vi "Chain3.vi"(7 "Name (\"\" to Use UUID)":string="CSM-Module") -> ()   [LabVIEW 2017, in "CSM-Testcase.lvlib"]
doc: "Creates a template for a CSM module without a user interface.\n\n> [!NOTE] CSM Name Rules\n> - The CSM module name must be unique to avoid entering the \"Critical Error\" state.\n> - If the input is \"\", a UUID will be used as the module name. This module will operate in independent mode and will not be listed in the module list.\n> - If the input ends with '#', the module will run in work mode. Modules with the same name will share the same message queue. External messages will be handled by the idle module.\n\n> [!NOTE] CSM Initialization State\n> - The default value is \"Macro: Initialize\", consistent with the JKISM state machine.\n> - This state is typically not modified and is provided to facilitate external programmatic changes to the initialization state.\n\n\n-- <b>Controls</b> --\n- <b>Name (\"\" to Use UUID)</b>: CSM Module Name\n- <b>Init State(\"Macro: Initialize\")</b>: Initialization State, default is \"Macro: Initialize\""
uses:
  CSM-Testcase.lvlib
  src/user.lib/_NEVSTOP/Communicable State Machine(CSM)/AdvanceAPI/CSM - Revert Arguments-Safe String.vi
  src/user.lib/_NEVSTOP/Communicable State Machine(CSM)/AdvanceAPI/CSM - Make String Arguments Safe.vi
  src/user.lib/_NEVSTOP/Communicable State Machine(CSM)/AdvanceAPI/CSM - Break Down Multiple States String.vi
  src/user.lib/_NEVSTOP/Communicable State Machine(CSM)/AdvanceAPI/CSM - Keywords.vi
  src/user.lib/_NEVSTOP/Communicable State Machine(CSM)/_Shared/Trim Single-line Text.vi
  Global-TestcaseCSM.vi
  src/user.lib/_NEVSTOP/Communicable State Machine(CSM)/_Polymophic/Build No-Reply Asynchronous Message with Arguments.vi
  src/user.lib/_NEVSTOP/Communicable State Machine(CSM)/_Polymophic/Build Asynchronous Message with Arguments.vi
  src/user.lib/_NEVSTOP/Communicable State Machine(CSM)/_Polymophic/Build Register Message.vi
  src/user.lib/_NEVSTOP/Communicable State Machine(CSM)/_Polymophic/Build Interrupt Broadcast Message.vi
  src/user.lib/_NEVSTOP/Communicable State Machine(CSM)/Communicable State Machine.lvlib
panel:
  out "Error Occurred":errorcluster
  out "State History":string
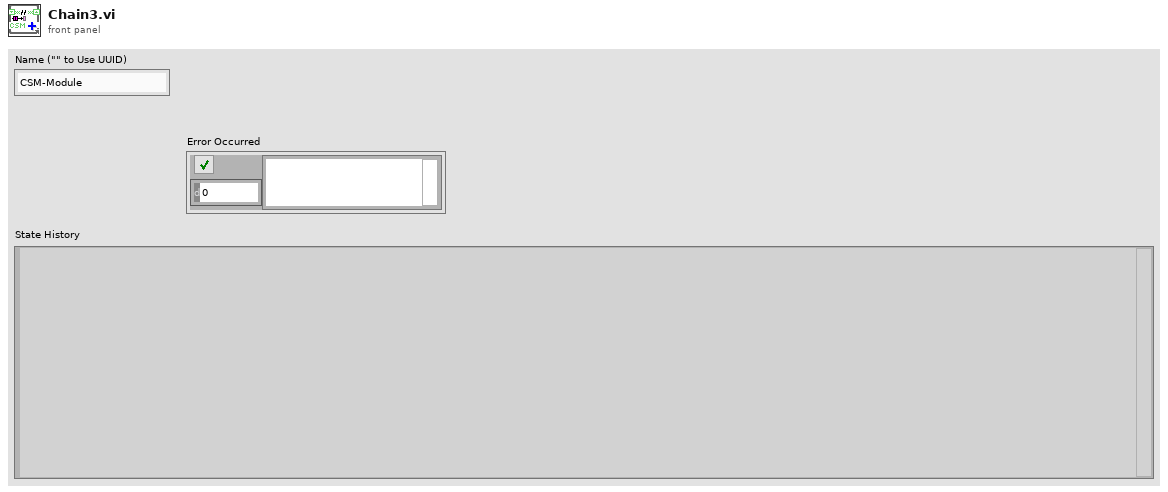
[diagram p1: front panel]
types:
  T1 = cluster{"Arguments":string, "Response":string, "error":errorcluster}
  T2 = enum32{"Invalid", "Standard", "Closed", "Hidden", "Minimized", "Maximized"}
  T3 = enum32{"invalid app kind", "Development System", "Run Time System", "Student Edition", "Embedded LabVIEW", "Evaluation", "Custom"}
  T4 = typedef "Communicable State Machine.lvlib/_CSM_Response Source Message.ctl" = cluster{"‘State":string, "’Arguments":string, "’Error":errorcluster}
  T5 = cluster{"Current VI Reference":refnum<vi>, "Close Panel on Exit?":bool}
  T6 = cluster{"Core":cluster{"Current VI Reference":refnum<vi>, "Close Panel on Exit?":bool}, "Your Boolean data":bool, "Your string data":string, "Counter":u32}
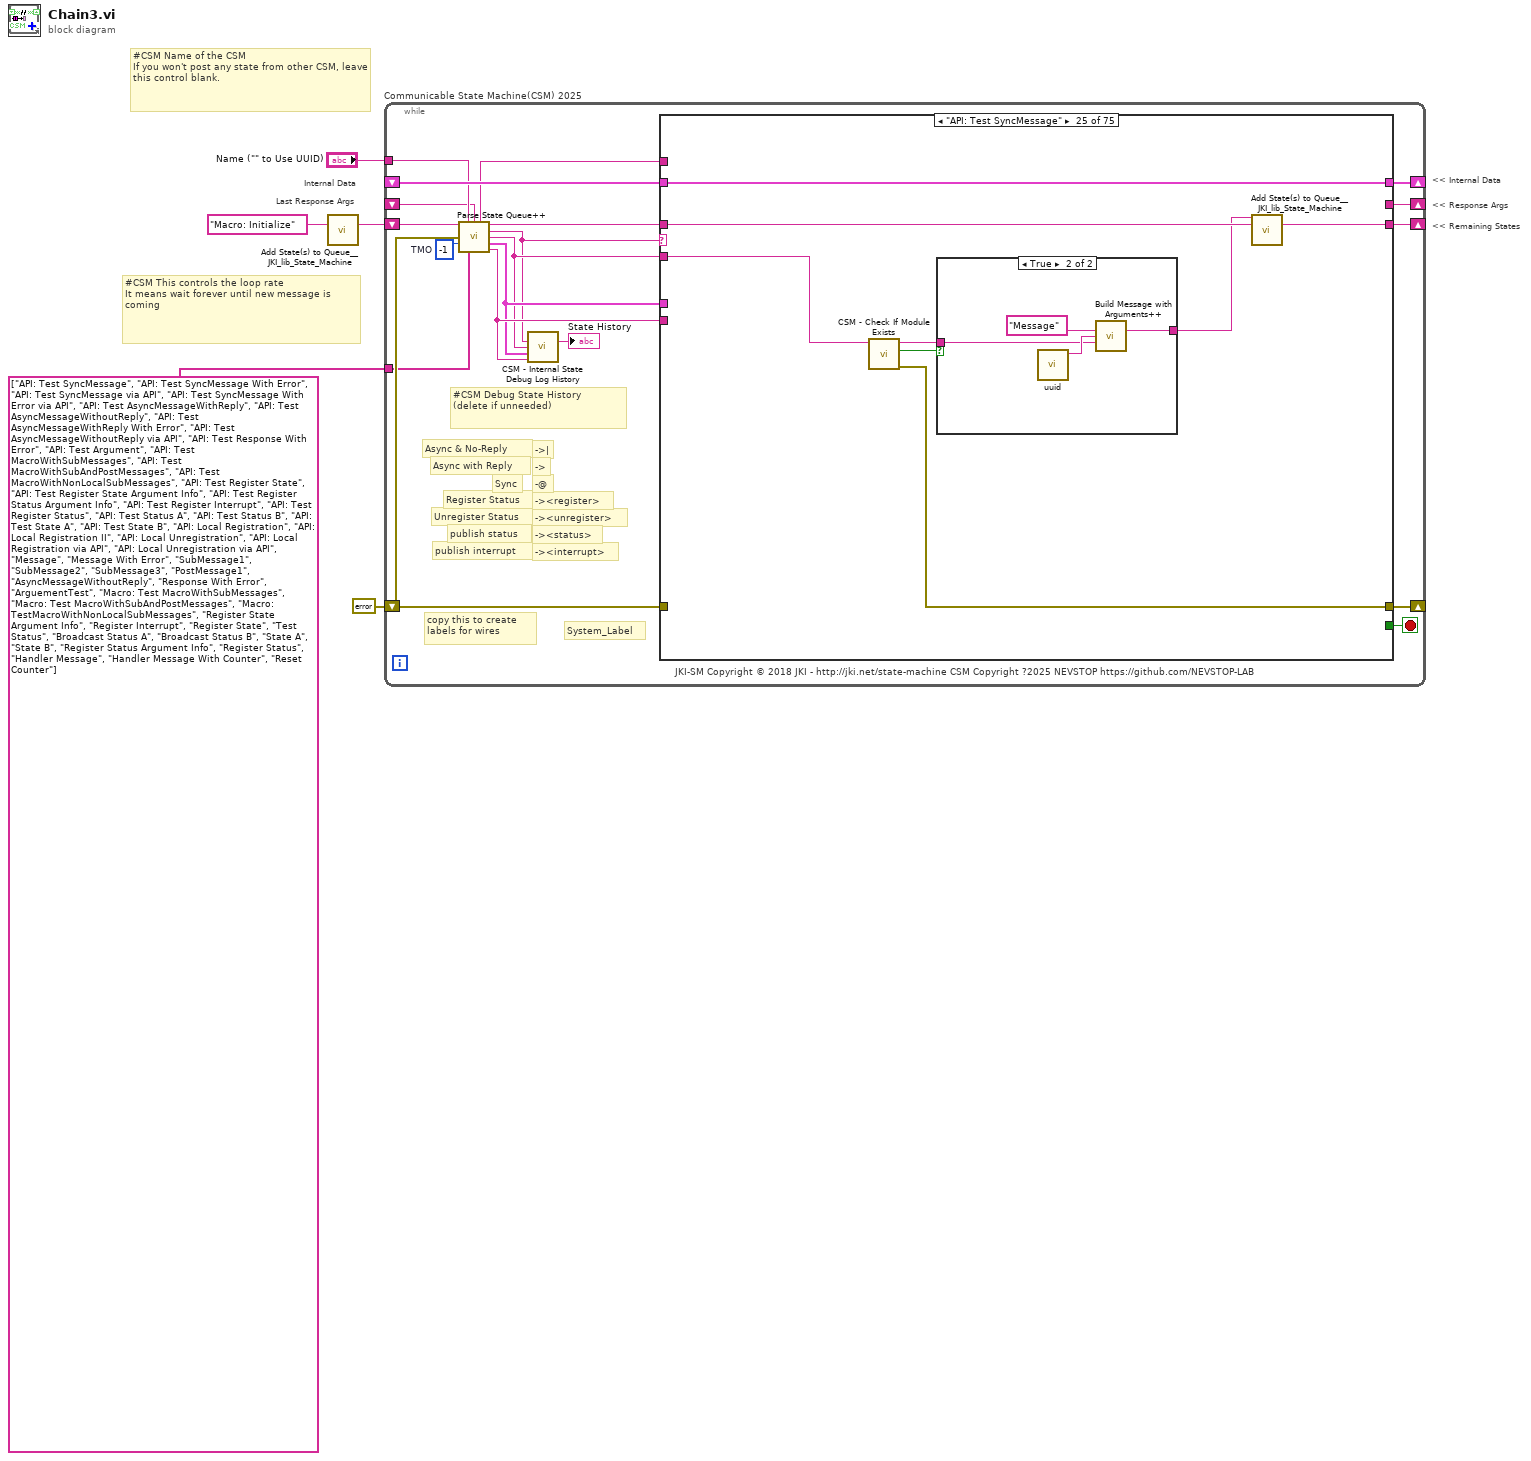
[diagram p0: block diagram]
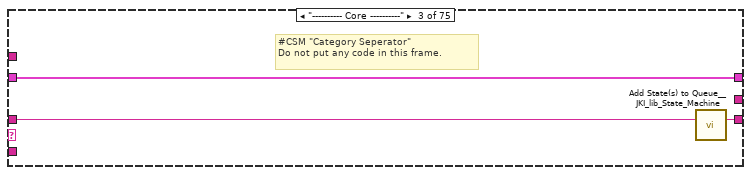
[diagram p4: hidden frame]
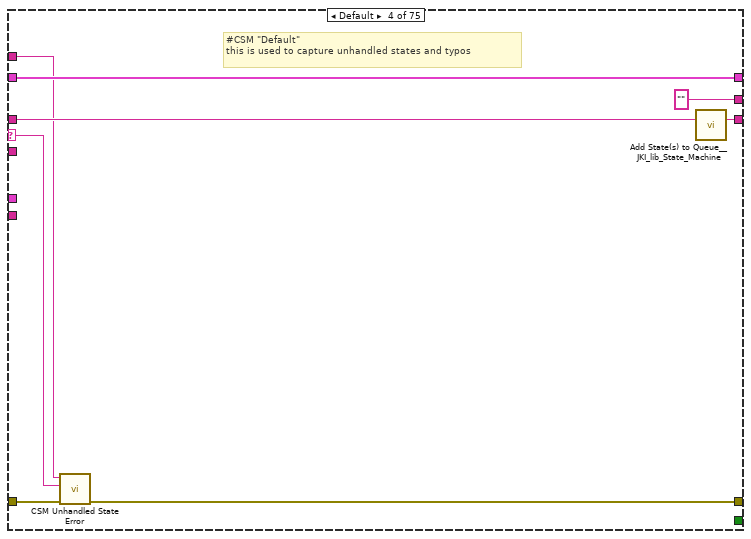
[diagram p5: hidden frame]
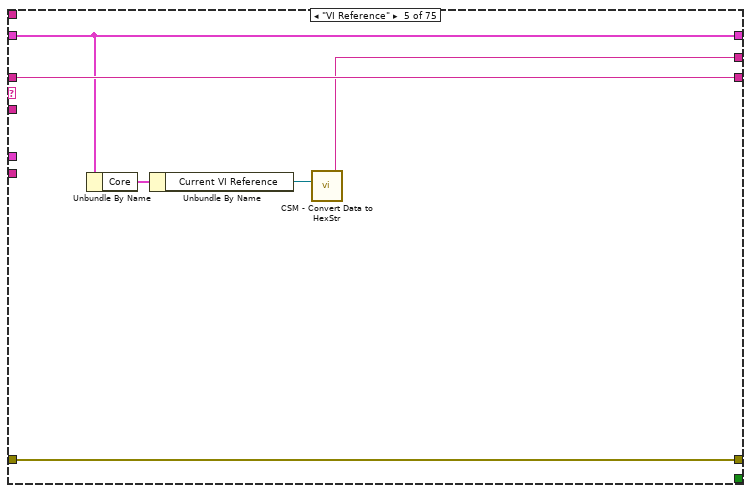
[diagram p6: hidden frame]
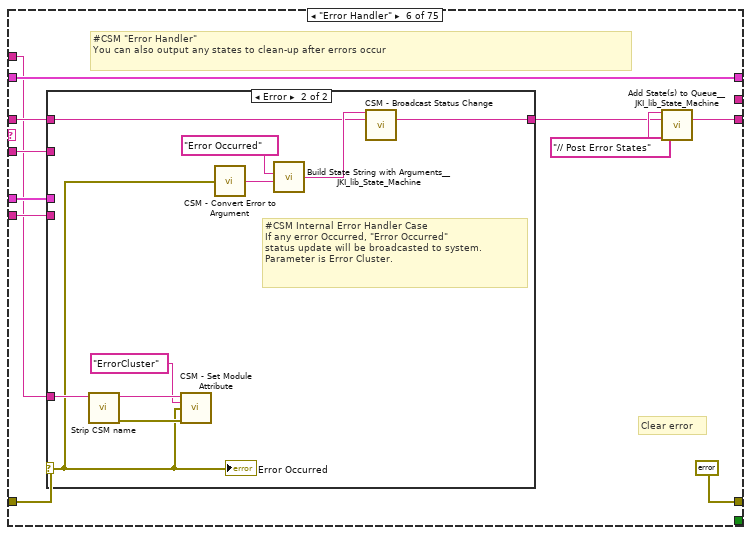
[diagram p7: hidden frame]
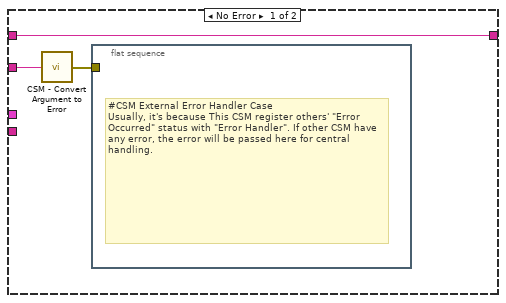
[diagram p8: hidden frame]
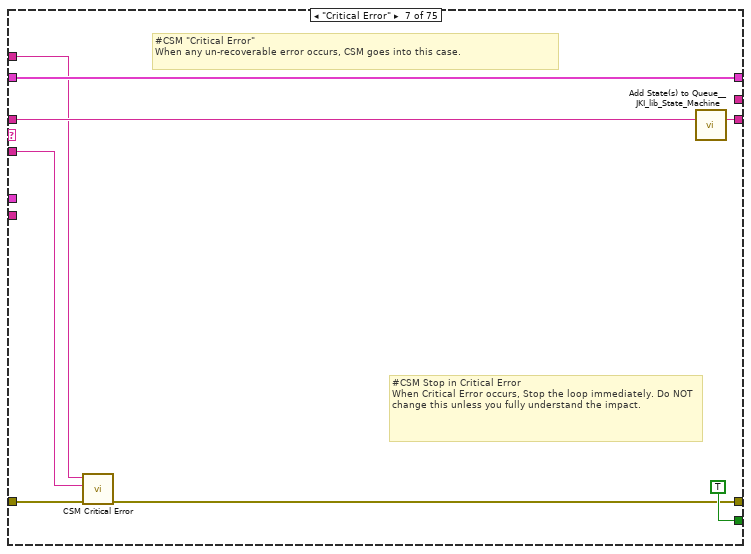
[diagram p9: hidden frame]
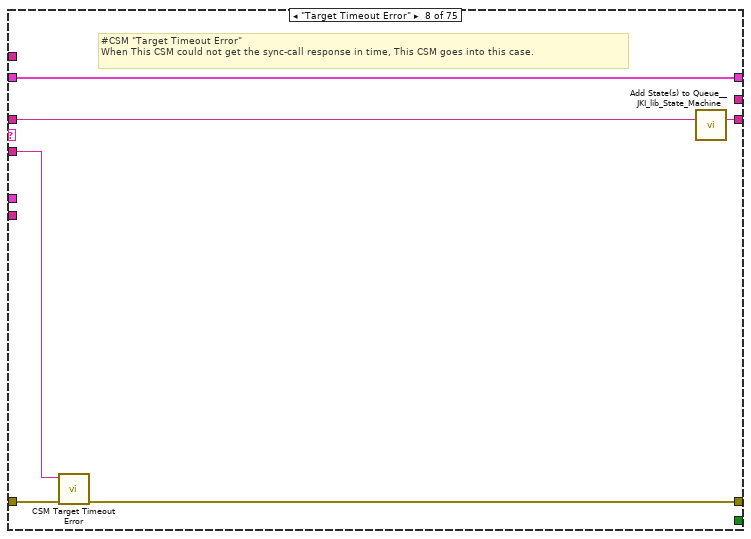
[diagram p10: hidden frame]
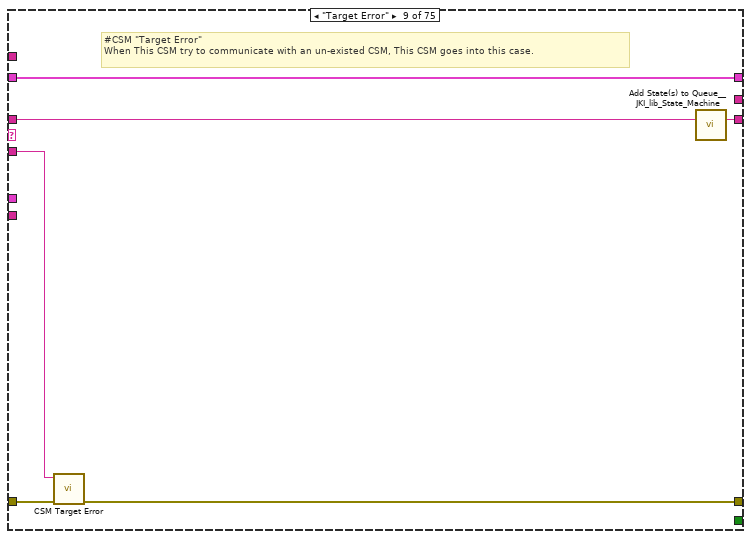
[diagram p11: hidden frame]
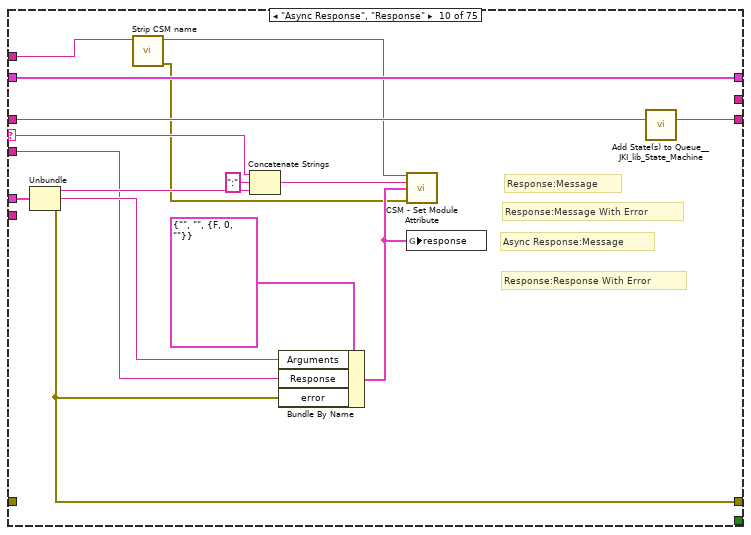
[diagram p12: hidden frame]
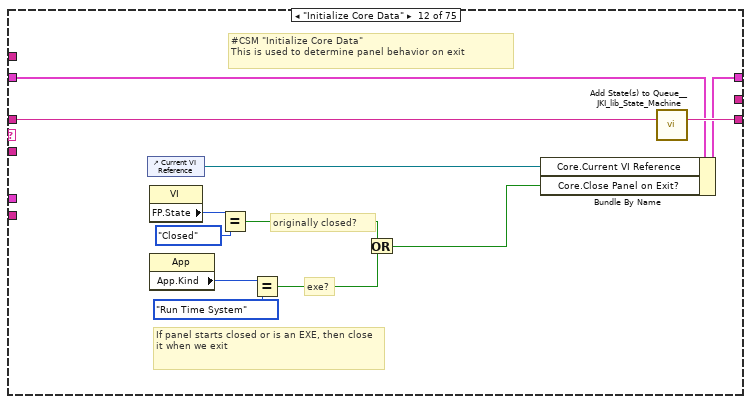
[diagram p14: hidden frame]
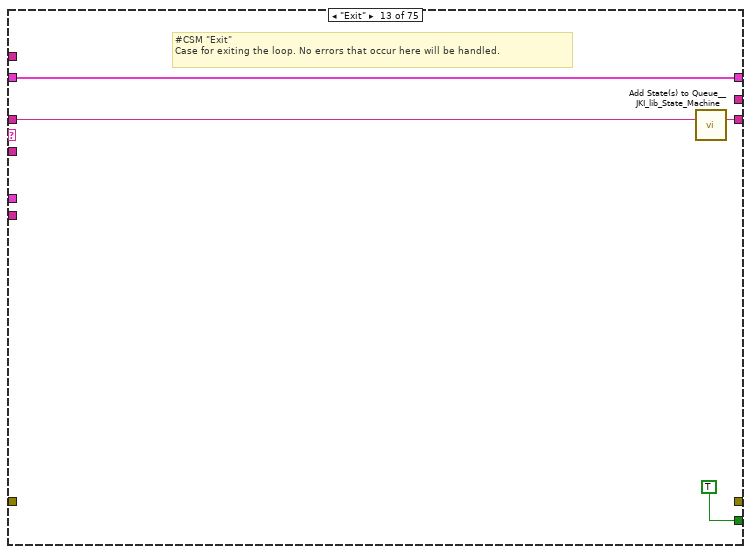
[diagram p15: hidden frame]
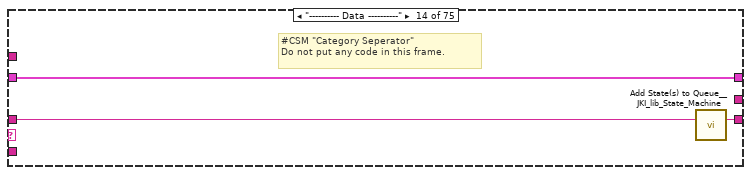
[diagram p16: hidden frame]
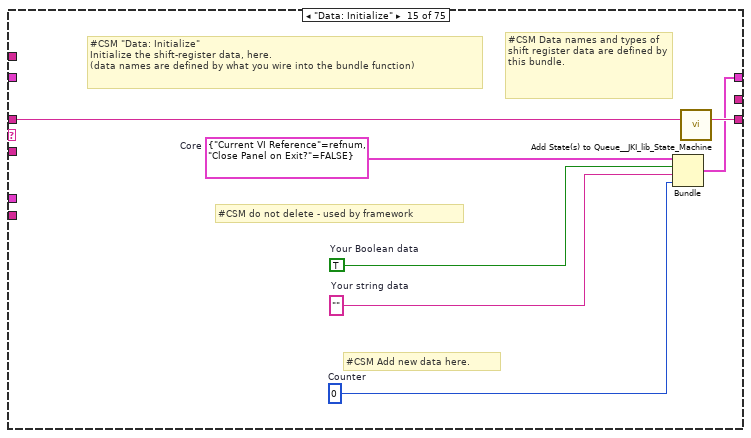
[diagram p17: hidden frame]
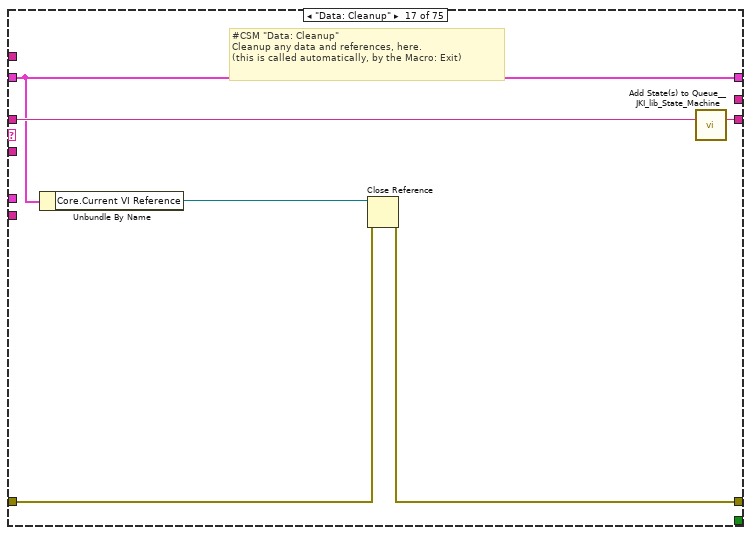
[diagram p19: hidden frame]
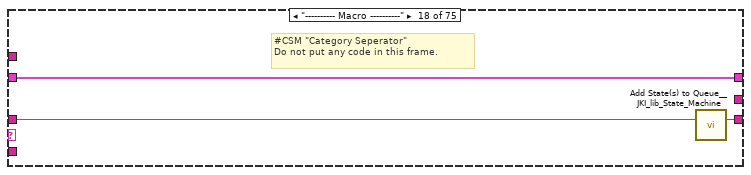
[diagram p20: hidden frame]
diagram:
  # "Last Response Args"
  # "Internal Data"
  # "#CSM Name of the CSM\nIf you won't post any state from other CSM, leave this control blank."
  # "#CSM This controls the loop rate\nIt means wait forever until new message is coming"
  # "<< Internal Data"
  # "<< Response Args"
  # "<< Remaining States"
  n1 = call <vilib>:"Add State(s) to Queue__JKI_lib_State_Machine.vi"("State(s) in (\"\")"="Macro: Initialize" ("Init State(\"Macro: Initialize\")")) -> ("States Out"=w5:string)  [unwired: 14 in]
  n2 = while "Communicable State Machine(CSM) 2025" {
    shift-right: [w19] -> _
    shift-left: _ -> [w18]
    shift-right: [w22] -> _
    shift-left: errorcluster {"status"=FALSE, "code"=0, "source"=""} ("error out") -> [w8]
    shift-right: [w21] -> _
    shift-left: w5 -> [w23]
    tunnel: "Name (\"\" to Use UUID)" -> [w15]
    shift-right: [w16] -> _
    shift-left: _ -> [w10]
    tunnel: string[] ["API: Test SyncMessage", "API: Test SyncMessage With Error", "API: Test SyncMessage via API", "API: Test SyncMessage With Error via API", "API: Test AsyncMessageWithReply", "API: Test AsyncMessageWithoutReply", "API: Test AsyncMessageWithReply With Error", "API: Test AsyncMessageWithoutReply via API", "API: Test Response With Error", "API: Test Argument", "API: Test MacroWithSubMessages", "API: Test MacroWithSubAndPostMessages", "API: Test MacroWithNonLocalSubMessages", "API: Test Register State", "API: Test Register State Argument Info", "API: Test Register Status Argument Info", "API: Test Register Interrupt", "API: Test Register Status", "API: Test Status A", "API: Test Status B", "API: Test State A", "API: Test State B", "API: Local Registration", "API: Local Registration II", "API: Local Unregistration", "API: Local Registration via API", "API: Local Unregistration via API", "Message", "Message With Error", "SubMessage1", "SubMessage2", "SubMessage3", "PostMessage1", "AsyncMessageWithoutReply", "Response With Error", "ArguementTest", "Macro: Test MacroWithSubMessages", "Macro: Test MacroWithSubAndPostMessages", "Macro: TestMacroWithNonLocalSubMessages", "Register State Argument Info", "Register Interrupt", "Register State", "Test Status", "Broadcast Status A", "Broadcast Status B", "State A", "State B", "Register Status Argument Info", "Register Status", "Handler Message", "Handler Message With Counter", "Reset Counter"] ("Allowed Messages (Empty for All)") -> [w6]
    stop <- w20 stop-if-true
    w17 = -1  # TMO
    # "#CSM Debug State History\n(delete if unneeded)"
    # "-><interrupt>"
    # "-><status>"
    # "-><unregister>"
    # "-><register>"
    # "-@"
    # "->"
    # "->|"
    # "publish interrupt"
    # "publish status"
    # "Unregister Status"
    # "Register Status"
    # "Sync"
    # "Async with Reply"
    # "Async & No-Reply"
    # "JKI-SM Copyright © 2018 JKI - http://jki.net/state-machine CSM Copyright ?2025 NEVSTOP https://github.com/NEVSTOP-LAB"
    # "copy this to create labels for wires"
    # "System_Label"
    n3 = call "Parse State Queue++.vi"("State Queue"=w23, "Name (\"\" to Use UUID)"=w15, "Response Arguments"=w10, "Previous Error"=w8, "Dequeue (1 ms)"=w17, "Allowed Messages (Empty for All)"=w6) -> ("Name Used"=w9:string, "Remaining States"=w24:string, "Current State"=w11:string, "Arguments"=w12:string, "Additional Information"=w13:T4, "Source CSM"=w14:string)  [unwired: 4 in]
    n4 = call "CSM - Internal State Debug Log History.vi"("State"=w11, "Arguments (\"\")"=w12, ">> Response Source Message >>"=w13, "Source (\"\")"=w14) -> ("Debug Log"=→"State History":string)  [unwired: 11 in]
    n5 = case shown="\"API: Test SyncMessage\"" w11 {
      selector: w11 -> [_ _ _ w35 _ _ _ _ _ w101 _ _ _ _ _ _ _ _ _ _ _ _ _ _ _ _ _ _ _ _ _ _ _ _ _ _ _ _ _ _ _ _ _ _ _ _ _ _ _ _ _ _ _ _ _ w543 _ _ _ _ _ _ _ _ _ _ w611 _ _ _ w636 w649 w656 w672 _]
      tunnel: w24 -> [w25 w28 w31 w39 w44 w50 w77 w83 w89 w105 w107 w119 w123 w126 w133 w135 w141 w144 w148 w154 w168 w188 w217 w221 w225 w237 w265 w297 w313 w325 w337 w351 w374 w385 w398 w405 w412 w419 w426 w433 w440 w447 w454 w461 w468 w475 w487 w496 w506 w516 w526 w530 w535 w538 w542 w549 w556 w559 w572 w578 w584 w588 w593 w597 w601 w605 w615 w619 w627 w633 w641 w651 w661 w677 w689]
      tunnel: w12 -> [_ _ _ _ _ w49 w73 w80 w86 w95 _ _ _ _ _ _ _ _ _ _ w155 w175 w200 _ w228 w240 w268 w300 w316 w328 w340 w354 w370 w388 w395 w402 w409 w416 w423 w430 w437 w444 w451 w458 w465 w472 w479 _ w498 w507 w517 w528 _ _ w539 _ w552 w561 _ w574 w580 w586 w591 w596 w600 w604 w610 w618 w625 w631 w638 w650 w655 w667 _]
      tunnel: w18 -> [w26 w27 w29 w37 w43 w55 w75 w81 w87 w103 w106 w113 w121 w124 _ w134 w136 w142 w146 w152 w170 w190 w219 w220 w229 w241 w269 w301 w317 w329 w341 w355 w377 w389 w400 w407 w414 w421 w428 w435 w442 w449 w456 w463 w470 w477 w485 w494 w504 w514 w524 w529 w533 w536 w540 w550 w557 w563 w573 w579 w585 w590 w595 w598 w602 w606 w616 w620 w626 w632 w642 w652 w662 w669 w687]
      tunnel: [_ _ _ w32 w45 errorcluster {"status"=FALSE, "code"=0, "source"=""} ("error out") w70 w78 w84 w94 _ _ _ _ _ _ w137 _ _ _ _ _ _ _ w222 w234 w262 w294 w310 w322 w334 w347 w371 w382 w399 w406 w413 w420 w427 w434 w441 w448 w455 w462 w469 w476 w481 w490 w500 w511 w521 _ _ _ _ w545 _ _ w565 _ _ w589 w594 w599 w603 w607 w609 w621 w622 w628 w635 w645 w657 w673 _] -> w22
      tunnel: w8 -> [_ _ _ w33 w45 w53 w71 w79 w85 _ _ _ _ _ _ _ w138 _ _ _ _ _ _ _ _ _ _ _ _ _ _ _ _ _ w399 w406 w413 w420 w427 w434 w441 w448 w455 w462 w469 w476 _ _ _ _ _ _ _ _ _ _ _ _ _ _ _ w589 w594 w599 w603 w607 w617 w621 w623 w629 w643 w653 w663 w678 _]
      tunnel: [w25 w28 w30 w38 w44 w51 w76 w82 w88 w104 w107 w118 w122 w125 w132 w135 w140 w143 w147 w153 w169 w189 w218 w221 w226 w238 w266 w298 w314 w326 w338 w352 w375 w386 w397 w404 w411 w418 w425 w432 w439 w446 w453 w460 w467 w474 w486 w495 w505 w515 w525 w530 w534 w537 w541 w551 w553 w558 w570 w575 w581 w587 w592 w597 w601 w605 w615 w619 w627 w633 w641 w651 w661 w677 w688] -> w21
      tunnel: [_ _ _ _ _ _ TRUE _ _ _ _ _ TRUE _ _ _ _ _ _ _ _ _ _ _ _ _ _ _ _ _ _ _ _ _ _ _ _ _ _ _ _ _ _ _ _ _ _ _ _ _ _ _ _ _ _ _ _ _ _ _ _ _ _ _ _ _ _ _ _ _ _ _ _ _ _] -> w20
      tunnel: [w26 w27 w29 w37 w43 w55 w75 w81 w87 w103 w106 w117 w121 w124 w131 w134 w136 w142 w146 w152 w170 w190 w219 w220 w229 w241 w269 w301 w317 w329 w341 w355 w377 w389 w400 w407 w414 w421 w428 w435 w442 w449 w456 w463 w470 w477 w485 w494 w504 w514 w524 w529 w533 w536 w540 w550 w557 w563 w573 w579 w585 w590 w595 w598 w602 w606 w616 w620 w626 w632 w642 w652 w662 w668 w685] -> w19
      tunnel: w14 -> [_ _ _ _ _ w48 _ _ _ _ _ _ _ _ _ _ _ _ _ _ _ _ _ _ _ _ _ _ _ _ _ _ _ _ _ _ _ _ _ _ _ _ _ _ _ _ _ _ _ _ _ _ _ _ _ _ _ _ _ _ _ _ _ _ _ _ _ _ _ _ _ _ _ _ _]
      tunnel: w13 -> [_ _ _ _ _ w47 _ _ _ w102 _ _ _ _ _ _ _ _ _ _ _ _ _ _ _ _ _ _ _ _ _ _ _ _ _ _ _ _ _ _ _ _ _ _ _ _ _ _ _ _ _ _ _ _ _ _ _ _ _ _ _ _ _ _ _ _ _ _ _ _ _ _ _ _ _]
      tunnel: [_ _ _ "" w40 _ _ _ _ _ _ _ _ _ _ _ _ _ _ _ _ _ _ _ _ _ _ _ _ _ _ _ _ _ _ _ _ _ _ _ _ _ _ _ _ _ _ _ _ _ _ w527 _ _ w539 w544 _ _ _ _ _ w586 w591 w596 w600 w604 w610 w618 w625 w631 _ w650 w655 _ _] -> w16
      tunnel: w9 -> [_ _ _ w34 _ w46 w72 _ _ w92 _ _ _ _ _ _ _ _ _ _ _ _ _ _ _ _ w253 w285 _ _ _ w348 _ _ _ _ _ _ _ _ _ _ _ _ _ _ w483 w492 w502 w513 w523 _ _ _ _ w546 _ _ w567 _ _ _ _ _ _ _ w614 _ _ _ w640 w648 w660 w676 _]
      frame "", "Idle" {
        # "#CSM \"Idle/Event Handler\"\nexecutes when the state queue is empty"
      }
      frame "CSM Documentation" {
        # "#CSM State Syntax\n\n// Comment line, all text to the right of “//” will be ignored\n// Local Message Example\nDoSth: DoA >> Arguments\n\n// Sync Call Example\nAPI: xxxx >> Arguments -@ TargetModule\n\n// Async Call Example\nAPI: xxxx >> Arguments -> TargetModule\n\n// Async Call without Reply Example\nAPI: xxxx >> Arguments ->| TargetModule\n\n// Broadcast normal status:\nStatus >> StatusArguments  -><status>\n\n// Broadcast Interrupt status:\nInterrupt >> StatusArguments  -><interrupt>\n\n// Register Source Module's status to Handler Module\nStatus@Source Module >> Handler Module@Handler Module -><register>\n\n// Unegister Source Module's status\nStatus@Source Module >> Handler Module -><unregister>"
        # "#CSM README FIRST\n\nCommunicable State Machine(CSM) is a LabVIEW application framework that builds upon JKI State Machine(JKISM). It follows the pattern of JKISM and extends the keywords to describe message communication between modules, including concepts such as Sync-Message, Async-Message, Subscription/Unsubscription of status - essential elements for creating reusable code modules. For more information, please visit the CSM wiki: https://nevstop-lab.github.io/CSM-Wiki/\n\nFor instructions on JKI State Machine, visit: \n    http://jki.net/state-machine/\nFor information about CSM, visit: \n    https://github.com/NEVSTOP-LAB"
        # "#CSM \"Documentation\"\nCase for holding CSM Documenation"
      }
      frame "---------- Core ----------" {
        # "#CSM \"Category Seperator\"\nDo not put any code in this frame."
        n6 = call <vilib>:"Add State(s) to Queue__JKI_lib_State_Machine.vi"("State(s) in (\"\")"=w31) -> ("States Out"=w30:string)  [unwired: 14 in]
      }
      frame Default {
        # "#CSM \"Default\"\nthis is used to capture unhandled states and typos"
        n7 = call "CSM Unhandled State Error.vi"("error in (no error)"=w33, "Undefined State"=w35, "CSM Name"=w34) -> ("error out"=w32:errorcluster)  [unwired: 8 in]
        n8 = call <vilib>:"Add State(s) to Queue__JKI_lib_State_Machine.vi"("State(s) in (\"\")"=w39) -> ("States Out"=w38:string)  [unwired: 14 in]
      }
      frame "VI Reference" {
        n9 = Unbundle By Name(w43) -> ("Core"=w42:T5)
        n10 = Unbundle By Name(w42) -> ("Current VI Reference"=w41:refnum<vi>)
        n11 = call "CSM - Convert Data to HexStr.vi"("Variant"=w41) -> ("HEX String (0-9,A-F)"=w40:string)  [unwired: 8 in]
      }
      frame "Error Handler" {
        # "#CSM \"Error Handler\"\nYou can also output any states to clean-up after errors occur"
        # "Clear error"
        n12 = case shown="Error" w53 {
          selector: w53 -> [_ w61]
          tunnel: [w59 w66] -> w52
          tunnel: w50 -> [w59 w65]
          tunnel: w49 -> [w58 _]
          tunnel: w48 -> [_ _]
          tunnel: w47 -> [_ _]
          tunnel: w46 -> [_ w64]
          frame No Error {
            n13 = call "CSM - Convert Argument to Error.vi"("Argument"=w58) -> ("Error"=w57:errorcluster)  [unwired: 4 in]
            n14 = flat-sequence {
              tunnel: w57 -> [_]
              frame #0 {
                # "#CSM External Error Handler Case\nUsually, it's because This CSM register others' \"Error Occurred\" status with \"Error Handler\". If other CSM have any error, the error will be passed here for central handling."
              }
            }
          }
          frame Error {
            # "#CSM Internal Error Handler Case \nIf any error Occurred, \"Error Occurred\" \nstatus update will be broadcasted to system.\nParameter is Error Cluster."
            n15 = call "Strip CSM name.vi"("CSM name"=w64) -> ("error out"=w63:errorcluster, "CSM name core"=w62:string)  [unwired: 7 in, 2 out]
            n16 = call "CSM - Set Module Attribute.vi"("CSM Name"=w62, "Attribute"="ErrorCluster", "Value"=w61, "Error In"=w63) -> ()  [unwired: 8 in, 4 out]
            n17 = call "CSM - Convert Error to Argument.vi"("Error"=w61) -> ("Argument"=w68:string)  [unwired: 4 in]
            n18 = call <vilib>:"Build State String with Arguments__JKI_lib_State_Machine.vi"("Arguments (\"\")"=w68, "State"="Error Occurred" ("Status with Arguments")) -> ("State with Arguments"=w67:string)  [unwired: 4 in]
            n19 = call "CSM - Broadcast Status Change.vi"("Status With Arguments"=w67, "State Queue"=w65) -> ("Remaining States"=w66:string)  [unwired: 13 in]
            "Error Occurred" <- w61
          }
        }
        n20 = call <vilib>:"Add State(s) to Queue__JKI_lib_State_Machine.vi"("State(s) in Front (\"\")"="// Post Error States", "State(s) in (\"\")"=w52) -> ("States Out"=w51:string)  [unwired: 13 in]
      }
      frame "Critical Error" {
        # "#CSM \"Critical Error\"\nWhen any un-recoverable error occurs, CSM goes into this case."
        # "#CSM Stop in Critical Error\nWhen Critical Error occurs, Stop the loop immediately. Do NOT change this unless you fully understand the impact."
        n21 = call "CSM Critical Error.vi"("error in (no error)"=w71, "Arugments (As Reason)"=w73, "CSM Name"=w72) -> ("error out"=w70:errorcluster)  [unwired: 8 in]
        n22 = call <vilib>:"Add State(s) to Queue__JKI_lib_State_Machine.vi"("State(s) in (\"\")"=w77) -> ("States Out"=w76:string)  [unwired: 14 in]
      }
      frame "Target Timeout Error" {
        # "#CSM \"Target Timeout Error\"\nWhen This CSM could not get the sync-call response in time, This CSM goes into this case."
        n23 = call "CSM Target Timeout Error.vi"("error in (no error)"=w79, "Arguments (As CSM Name)"=w80) -> ("error out"=w78:errorcluster)  [unwired: 9 in]
        n24 = call <vilib>:"Add State(s) to Queue__JKI_lib_State_Machine.vi"("State(s) in (\"\")"=w83) -> ("States Out"=w82:string)  [unwired: 14 in]
      }
      frame "Target Error" {
        # "#CSM \"Target Error\"\nWhen This CSM try to communicate with an un-existed CSM, This CSM goes into this case."
        n25 = call "CSM Target Error.vi"("error in (no error)"=w85, "Arguments (As CSM Name)"=w86) -> ("error out"=w84:errorcluster)  [unwired: 9 in]
        n26 = call <vilib>:"Add State(s) to Queue__JKI_lib_State_Machine.vi"("State(s) in (\"\")"=w89) -> ("States Out"=w88:string)  [unwired: 14 in]
      }
      frame "Async Response", "Response" {
        # "Response:Response With Error"
        # "Response:Message With Error"
        # "Async Response:Message"
        # "Response:Message"
        n27 = Unbundle(w102) -> ("‘State"=w100:string, "’Arguments"=w96:string, "’Error"=w94:errorcluster)
        n28 = call "Strip CSM name.vi"("CSM name"=w92) -> ("error out"=w90:errorcluster, "CSM name core"=w91:string)  [unwired: 7 in, 2 out]
        n29 = Concatenate Strings(w101, ":" ("string"), w100) -> (w98:string)
        n30 = Bundle By Name(cluster=T1 {"Arguments"="", "Response"="", "error"={"status"=FALSE, "code"=0, "source"=""}}, "Arguments"=w96, "Response"=w95, "error"=w94) -> (w93:T1)
        n31 = call "CSM - Set Module Attribute.vi"("CSM Name"=w91, "Attribute"=w98, "Value"=w93, "Error In"=w90) -> ()  [unwired: 8 in, 4 out]
        n32 = global write "Global-TestcaseCSM.vi" "response"(w93) -> ()
        n33 = call <vilib>:"Add State(s) to Queue__JKI_lib_State_Machine.vi"("State(s) in (\"\")"=w105) -> ("States Out"=w104:string)  [unwired: 14 in]
      }
      frame "Async Message Posted" {
        # "#CSM \"Async Message Posted\"\nAfter Async Message is posted (-> or ->| ), CSM goes to this state for post-action.\nYou can use Argument - State to tell which Async Message is called."
      }
      frame "Initialize Core Data" {
        # "#CSM \"Initialize Core Data\"\nThis is used to determine panel behavior on exit"
        # "originally closed?"
        # "exe?"
        # "If panel starts closed or is an EXE, then close it when we exit"
        n34 = control-ref of="Current VI Reference"() -> (w111:refnum<vi>)
        n35 = property class="VI"() -> ("FP.State"=w110:T2)  [unwired: 2 in, 2 out]
        n36 = property class="App"() -> ("App.Kind"=w116:T3)  [unwired: 2 in, 2 out]
        n37 = Equal?(x=w110, y=T2."Closed" ("Front Panel Window:State")) -> (x = y?=w108:bool)
        n38 = Equal?(x=w116, y=T3."Run Time System" ("Application:Kind")) -> (x = y?=w114:bool)
        n39 = Or(x=w108, y=w114) -> (x .or. y?=w112:bool)
        n40 = Bundle By Name(cluster=w113, "Core.Current VI Reference"=w111, "Core.Close Panel on Exit?"=w112) -> (w117:T6)
        n41 = call <vilib>:"Add State(s) to Queue__JKI_lib_State_Machine.vi"("State(s) in (\"\")"=w119) -> ("States Out"=w118:string)  [unwired: 14 in]
      }
      frame "Exit" {
        # "#CSM \"Exit\"\nCase for exiting the loop. No errors that occur here will be handled."
        n42 = call <vilib>:"Add State(s) to Queue__JKI_lib_State_Machine.vi"("State(s) in (\"\")"=w123) -> ("States Out"=w122:string)  [unwired: 14 in]
      }
      frame "---------- Data ----------" {
        # "#CSM \"Category Seperator\"\nDo not put any code in this frame."
        n43 = call <vilib>:"Add State(s) to Queue__JKI_lib_State_Machine.vi"("State(s) in (\"\")"=w126) -> ("States Out"=w125:string)  [unwired: 14 in]
      }
      frame "Data: Initialize" {
        w127 = u32 0  # Counter
        w128 = T5 {"Current VI Reference"=refnum, "Close Panel on Exit?"=FALSE}  # Core
        w130 = TRUE  # Your Boolean data
        w129 = ""  # Your string data
        # "#CSM \"Data: Initialize\"\nInitialize the shift-register data, here.\n(data names are defined by what you wire into the bundle function)"
        # "#CSM do not delete - used by framework"
        # "#CSM Add new data here."
        # "#CSM Data names and types of shift register data are defined by this bundle."
        n44 = Bundle("Core"=w128, "Your Boolean data"=w130, "Your string data"=w129, "Counter"=w127) -> (w131:T6)  [unwired: 1 in]
        n45 = call <vilib>:"Add State(s) to Queue__JKI_lib_State_Machine.vi"("State(s) in (\"\")"=w133) -> ("States Out"=w132:string)  [unwired: 14 in]
      }
      frame "Data: Update Indicators" {
      }
      frame "Data: Cleanup" {
        # "#CSM \"Data: Cleanup\"\nCleanup any data and references, here.\n(this is called automatically, by the Macro: Exit)"
        n46 = Unbundle By Name(w136) -> ("Core.Current VI Reference"=w139:refnum<vi>)
        n47 = Close Reference(reference=w139, error in (no error)=w138) -> (error out=w137:errorcluster)
        n48 = call <vilib>:"Add State(s) to Queue__JKI_lib_State_Machine.vi"("State(s) in (\"\")"=w141) -> ("States Out"=w140:string)  [unwired: 14 in]
      }
      frame "---------- Macro ----------" {
        # "#CSM \"Category Seperator\"\nDo not put any code in this frame."
        n49 = call <vilib>:"Add State(s) to Queue__JKI_lib_State_Machine.vi"("State(s) in (\"\")"=w144) -> ("States Out"=w143:string)  [unwired: 14 in]
      }
      frame "Macro: Initialize" {
        # "#CSM \"Macro: Initialize\"\nInitialization Macro (This is called once, when the VI starts)"
        n50 = call <vilib>:"Add State(s) to Queue__JKI_lib_State_Machine.vi"("State(s) in Front (\"\")"="Data: Initialize\nInitialize Core Data\nData: Update Indicators", "State(s) in (\"\")"=w148) -> ("States Out"=w147:string)  [unwired: 13 in]
      }
      frame "Macro: Exit" {
        # "#CSM \"Macro: Exit\"\nExit Macro (This is called once, when the VI exits)"
        n51 = call <vilib>:"Add State(s) to Queue__JKI_lib_State_Machine.vi"("State(s) in Front (\"\")"="//Exit Sub-Modules ", "State(s) at Back (\"\")"="Data: Cleanup\nExit") -> ("States Out"=w150:string)  [unwired: 13 in]
        n52 = call <vilib>:"Add State(s) to Queue__JKI_lib_State_Machine.vi"("State(s) in Front (\"\")"=w150, "State(s) in (\"\")"=w154) -> ("States Out"=w153:string)  [unwired: 13 in]
      }
      frame "Macro: Test MacroWithSubMessages" {
        w156 = "SubMessage2" ("State With Arguments")
        w158 = "SubMessage1" ("State With Arguments")
        n53 = call "uuid.vi"() -> ("UUID"=w157:string)  [unwired: 11 in]
        n54 = call "uuid.vi"() -> ("UUID"=w159:string)  [unwired: 11 in]
        n55 = Concatenate Strings(w158, w159) -> (w160:string)
        n56 = Concatenate Strings(w156, w157) -> (w161:string)
        n57 = call <vilib>:"Build State String with Arguments__JKI_lib_State_Machine.vi"("Arguments (\"\")"=w155, "State"="SubMessage3" ("State With Arguments")) -> ("State with Arguments"=w163:string)  [unwired: 4 in]
        n58 = call <vilib>:"Build State String with Arguments__JKI_lib_State_Machine.vi"("Arguments (\"\")"=w160, "State"=w158) -> ("State with Arguments"=w165:string)  [unwired: 4 in]
        n59 = call <vilib>:"Build State String with Arguments__JKI_lib_State_Machine.vi"("Arguments (\"\")"=w161, "State"=w156) -> ("State with Arguments"=w164:string)  [unwired: 4 in]
        n60 = Build Array(w165, w164, w163) -> (w162:string[])
        n61 = call "CSM - Compact Multiple States.vi"("Multiple States"=w162) -> ("States"=w167:string)  [unwired: 9 in]
        n62 = call <vilib>:"Add State(s) to Queue__JKI_lib_State_Machine.vi"("State(s) in Front (\"\")"=w167, "State(s) in (\"\")"=w168) -> ("States Out"=w169:string)  [unwired: 13 in]
      }
      frame "Macro: Test MacroWithSubAndPostMessages" {
        w174 = "PostMessage1" ("State With Arguments")
        w176 = "SubMessage2" ("State With Arguments")
        w178 = "SubMessage1" ("State With Arguments")
        n63 = call "uuid.vi"() -> ("UUID"=w177:string)  [unwired: 11 in]
        n64 = call "uuid.vi"() -> ("UUID"=w173:string)  [unwired: 11 in]
        n65 = call "uuid.vi"() -> ("UUID"=w179:string)  [unwired: 11 in]
        n66 = Concatenate Strings(w174, w173) -> (w172:string)
        n67 = Concatenate Strings(w178, w179) -> (w180:string)
        n68 = Concatenate Strings(w176, w177) -> (w181:string)
        n69 = call <vilib>:"Build State String with Arguments__JKI_lib_State_Machine.vi"("Arguments (\"\")"=w175, "State"="SubMessage3" ("State With Arguments")) -> ("State with Arguments"=w183:string)  [unwired: 4 in]
        n70 = call <vilib>:"Build State String with Arguments__JKI_lib_State_Machine.vi"("Arguments (\"\")"=w172, "State"=w174) -> ("State with Arguments"=w171:string)  [unwired: 4 in]
        n71 = call <vilib>:"Build State String with Arguments__JKI_lib_State_Machine.vi"("Arguments (\"\")"=w180, "State"=w178) -> ("State with Arguments"=w185:string)  [unwired: 4 in]
        n72 = call <vilib>:"Build State String with Arguments__JKI_lib_State_Machine.vi"("Arguments (\"\")"=w181, "State"=w176) -> ("State with Arguments"=w184:string)  [unwired: 4 in]
        n73 = Build Array(w185, w184, w183) -> (w182:string[])
        n74 = call "CSM - Compact Multiple States.vi"("Multiple States"=w182) -> ("States"=w187:string)  [unwired: 9 in]
        n75 = call <vilib>:"Add State(s) to Queue__JKI_lib_State_Machine.vi"("State(s) in Front (\"\")"=w187, "State(s) in (\"\")"=w188, "State(s) at Back (\"\")"=w171) -> ("States Out"=w189:string)  [unwired: 12 in]
      }
      frame "Macro: TestMacroWithNonLocalSubMessages" {
        w204 = "PostMessage1" ("State With Arguments")
        w205 = "SubMessage2" ("State With Arguments")
        w207 = "SubMessage1" ("State With Arguments")
        n76 = Match Pattern(string=w200, regular expression="+") -> (before substring=w192:string, after substring=w191:string)  [unwired: 1 in, 2 out]
        n77 = call "uuid.vi"() -> ("UUID"=w203:string)  [unwired: 11 in]
        n78 = call "uuid.vi"() -> ("UUID"=w206:string)  [unwired: 11 in]
        n79 = call "uuid.vi"() -> ("UUID"=w208:string)  [unwired: 11 in]
        n80 = Concatenate Strings(w204, w203) -> (w202:string)
        n81 = Concatenate Strings(w207, w208) -> (w209:string)
        n82 = Concatenate Strings(w205, w206) -> (w210:string)
        n83 = call <vilib>:"Build State String with Arguments__JKI_lib_State_Machine.vi"("Arguments (\"\")"=w202, "State"=w204) -> ("State with Arguments"=w201:string)  [unwired: 4 in]
        n84 = call-poly "Build Message with Arguments++.vi"("State With Arguments"="SubMessage1", "Target Module (\"\")"=w191) -> ("CSM Message String"=w196:string)  [unwired: 13 in]
        n85 = call-poly "Build Message with Arguments++.vi"("State With Arguments"="SubMessage2", "Target Module (\"\")"=w191) -> ("CSM Message String"=w195:string)  [unwired: 13 in]
        n86 = call <vilib>:"Build State String with Arguments__JKI_lib_State_Machine.vi"("Arguments (\"\")"=w192, "State"="SubMessage3" ("State With Arguments")) -> ("State with Arguments"=w212:string)  [unwired: 4 in]
        n87 = call-poly "Build Message with Arguments++.vi"("State With Arguments"="Message", "Target Module (\"\")"=w191) -> ("CSM Message String"=w197:string)  [unwired: 13 in]
        n88 = call <vilib>:"Build State String with Arguments__JKI_lib_State_Machine.vi"("Arguments (\"\")"=w209, "State"=w207) -> ("State with Arguments"=w214:string)  [unwired: 4 in]
        n89 = call <vilib>:"Build State String with Arguments__JKI_lib_State_Machine.vi"("Arguments (\"\")"=w210, "State"=w205) -> ("State with Arguments"=w213:string)  [unwired: 4 in]
        n90 = Build Array(w214, w213, w212, w197, w196, w195) -> (w211:string[])
        n91 = call "CSM - Compact Multiple States.vi"("Multiple States"=w211) -> ("States"=w216:string)  [unwired: 9 in]
        n92 = call <vilib>:"Add State(s) to Queue__JKI_lib_State_Machine.vi"("State(s) in Front (\"\")"=w216, "State(s) in (\"\")"=w217, "State(s) at Back (\"\")"=w201) -> ("States Out"=w218:string)  [unwired: 12 in]
      }
      frame "---------- API ----------" {
        # "#CSM \"Category Seperator\"\nDo not put any code in this frame."
      }
      frame "API: Test SyncMessage" {
        n93 = call "CSM - Check If Module Exists.vi"("CSM Name"=w228) -> ("error out"=w222:errorcluster, "Exist?"=w223:bool, "CSM Name (Dup)"=w227:string)  [unwired: 8 in]
        n94 = case shown="True" w223 {
          tunnel: w227 -> [_ w231]
          tunnel: [_ w230] -> w224
          frame False {
          }
          frame True {
            n95 = call "uuid.vi"() -> ("UUID"=w232:string)  [unwired: 11 in]
            n96 = call-poly "Build Message with Arguments++.vi"("State With Arguments"="Message", "Arguments (\"\")"=w232, "Target Module (\"\")"=w231) -> ("CSM Message String"=w230:string)  [unwired: 12 in]
          }
        }
        n97 = call <vilib>:"Add State(s) to Queue__JKI_lib_State_Machine.vi"("State(s) in Front (\"\")"=w224, "State(s) in (\"\")"=w225) -> ("States Out"=w226:string)  [unwired: 13 in]
      }
      frame "API: Test SyncMessage With Error" {
        n98 = call "CSM - Check If Module Exists.vi"("CSM Name"=w240) -> ("error out"=w234:errorcluster, "Exist?"=w235:bool, "CSM Name (Dup)"=w239:string)  [unwired: 8 in]
        n99 = case shown="True" w235 {
          tunnel: w239 -> [_ w243]
          tunnel: [_ w242] -> w236
          frame False {
          }
          frame True {
            n100 = call "uuid.vi"() -> ("UUID"=w244:string)  [unwired: 11 in]
            n101 = call "Build Synchronous Message with Arguments.vi"("State With Arguments"="Message With Error", "Arguments (\"\")"=w244, "Target Module (\"\")"=w243) -> ("CSM Message String"=w242:string)  [unwired: 12 in]
          }
        }
        n102 = call <vilib>:"Add State(s) to Queue__JKI_lib_State_Machine.vi"("State(s) in Front (\"\")"=w236, "State(s) in (\"\")"=w237) -> ("States Out"=w238:string)  [unwired: 13 in]
      }
      frame "API: Test SyncMessage via API" {
        n103 = call "CSM - Check If Module Exists.vi"("CSM Name"=w268) -> ("error out"=w263:errorcluster, "Exist?"=w264:bool, "CSM Name (Dup)"=w267:string)  [unwired: 8 in]
        n104 = case shown="True" w264 {
          tunnel: w267 -> [_ w277]
          tunnel: [_ w276] -> w251
          tunnel: w253 -> [_ w275]
          tunnel: [_ w274] -> w260
          tunnel: [_ w273] -> w249
          tunnel: [_ w272] -> w256
          tunnel: [_ w271] -> w259
          frame False {
          }
          frame True {
            w274 = "Message" ("State With Arguments")
            n105 = call "uuid.vi"() -> ("UUID"=w272:string)  [unwired: 11 in]
            n106 = call "CSM - Wait and Send Message for Reply.vi"("State"=w274, "Current Module (\"\" to Generate an ID)"=w275, "Arguments (\"\")"=w272, "Target Module"=w277) -> ("Response"=w271:string, "Source CSM"=w273:string, "error out"=w276:errorcluster)  [unwired: 9 in]
          }
        }
        n107 = call "Strip CSM name.vi"("CSM name"=w253) -> ("error out"=w250:errorcluster, "CSM name core"=w252:string)  [unwired: 7 in, 2 out]
        n108 = call "Strip CSM name.vi"("CSM name"=w249) -> ("error out"=w246:errorcluster, "CSM name core"=w248:string)  [unwired: 7 in, 2 out]
        n109 = Bundle By Name(cluster=T1 {"Arguments"="", "Response"="", "error"={"status"=FALSE, "code"=0, "source"=""}}, "Arguments"=w256, "Response"=w259, "error"=w251) -> (w254:T1)
        n110 = Concatenate Strings(w248, ":" ("string"), w260) -> (w258:string)
        n111 = Merge Errors(w250, w246) -> (w247:errorcluster)
        n112 = call "CSM - Set Module Attribute.vi"("CSM Name"=w252, "Attribute"=w258, "Value"=w254, "Error In"=w247) -> ("error out"=w257:errorcluster)  [unwired: 8 in, 3 out]
        n113 = disable-structure shown="Enabled" {
          disable-tunnel: w254 -> [w270 _]
          frame Enabled {
            n114 = global write "Global-TestcaseCSM.vi" "response"(w270) -> ()
          }
          frame Disabled {
          }
        }
        n115 = call <vilib>:"Add State(s) to Queue__JKI_lib_State_Machine.vi"("State(s) in (\"\")"=w265) -> ("States Out"=w266:string)  [unwired: 14 in]
        n116 = Merge Errors(w257, w251, w263) -> (w262:errorcluster)
      }
      frame "API: Test SyncMessage With Error via API" {
        n117 = call "CSM - Check If Module Exists.vi"("CSM Name"=w300) -> ("error out"=w295:errorcluster, "Exist?"=w296:bool, "CSM Name (Dup)"=w299:string)  [unwired: 8 in]
        n118 = case shown="True" w296 {
          tunnel: w299 -> [_ w309]
          tunnel: [_ w308] -> w282
          tunnel: w285 -> [_ w307]
          tunnel: [_ w306] -> w292
          tunnel: [_ w305] -> w281
          tunnel: [_ w304] -> w288
          tunnel: [_ w303] -> w291
          frame False {
          }
          frame True {
            w306 = "Message With Error" ("State With Arguments")
            n119 = call "uuid.vi"() -> ("UUID"=w304:string)  [unwired: 11 in]
            n120 = call "CSM - Wait and Send Message for Reply.vi"("State"=w306, "Current Module (\"\" to Generate an ID)"=w307, "Arguments (\"\")"=w304, "Target Module"=w309) -> ("Response"=w303:string, "Source CSM"=w305:string, "error out"=w308:errorcluster)  [unwired: 9 in]
          }
        }
        n121 = call "Strip CSM name.vi"("CSM name"=w281) -> ("error out"=w278:errorcluster, "CSM name core"=w280:string)  [unwired: 7 in, 2 out]
        n122 = Bundle By Name(cluster=T1 {"Arguments"="", "Response"="", "error"={"status"=FALSE, "code"=0, "source"=""}}, "Arguments"=w288, "Response"=w291, "error"=w282) -> (w287:T1)
        n123 = call "Strip CSM name.vi"("CSM name"=w285) -> ("error out"=w283:errorcluster, "CSM name core"=w284:string)  [unwired: 7 in, 2 out]
        n124 = Concatenate Strings(w280, ":" ("string"), w292) -> (w290:string)
        n125 = Merge Errors(w283, w278) -> (w279:errorcluster)
        n126 = disable-structure shown="Enabled" {
          disable-tunnel: w287 -> [w302 _]
          frame Enabled {
            n127 = global write "Global-TestcaseCSM.vi" "response"(w302) -> ()
          }
          frame Disabled {
          }
        }
        n128 = call "CSM - Set Module Attribute.vi"("CSM Name"=w284, "Attribute"=w290, "Value"=w287, "Error In"=w279) -> ("error out"=w289:errorcluster)  [unwired: 8 in, 3 out]
        n129 = call <vilib>:"Add State(s) to Queue__JKI_lib_State_Machine.vi"("State(s) in (\"\")"=w297) -> ("States Out"=w298:string)  [unwired: 14 in]
        n130 = Merge Errors(w289, w282, w295) -> (w294:errorcluster)
      }
      frame "API: Test AsyncMessageWithReply" {
        n131 = call "CSM - Check If Module Exists.vi"("CSM Name"=w316) -> ("error out"=w310:errorcluster, "Exist?"=w311:bool, "CSM Name (Dup)"=w315:string)  [unwired: 8 in]
        n132 = case shown="True" w311 {
          tunnel: w315 -> [_ w319]
          tunnel: [_ w318] -> w312
          frame False {
          }
          frame True {
            n133 = call "uuid.vi"() -> ("UUID"=w320:string)  [unwired: 11 in]
            n134 = call-poly "Build Message with Arguments++.vi"("State With Arguments"="Message", "Arguments (\"\")"=w320, "Target Module (\"\")"=w319) -> ("CSM Message String"=w318:string)  [unwired: 12 in]
          }
        }
        n135 = call <vilib>:"Add State(s) to Queue__JKI_lib_State_Machine.vi"("State(s) in Front (\"\")"=w312, "State(s) in (\"\")"=w313) -> ("States Out"=w314:string)  [unwired: 13 in]
      }
      frame "API: Test AsyncMessageWithReply With Error" {
        n136 = call "CSM - Check If Module Exists.vi"("CSM Name"=w328) -> ("error out"=w322:errorcluster, "Exist?"=w323:bool, "CSM Name (Dup)"=w327:string)  [unwired: 8 in]
        n137 = case shown="True" w323 {
          tunnel: w327 -> [_ w332]
          tunnel: [_ w330] -> w324
          frame False {
          }
          frame True {
            n138 = call "uuid.vi"() -> ("UUID"=w331:string)  [unwired: 11 in]
            n139 = call-poly "Build Message with Arguments++.vi"("State With Arguments"="Message With Error", "Arguments (\"\")"=w331, "Target Module (\"\")"=w332) -> ("CSM Message String"=w330:string)  [unwired: 12 in]
          }
        }
        n140 = call <vilib>:"Add State(s) to Queue__JKI_lib_State_Machine.vi"("State(s) in Front (\"\")"=w324, "State(s) in (\"\")"=w325) -> ("States Out"=w326:string)  [unwired: 13 in]
      }
      frame "API: Test AsyncMessageWithoutReply" {
        n141 = call "CSM - Check If Module Exists.vi"("CSM Name"=w340) -> ("error out"=w334:errorcluster, "Exist?"=w335:bool, "CSM Name (Dup)"=w339:string)  [unwired: 8 in]
        n142 = case shown="True" w335 {
          tunnel: w339 -> [_ w345]
          tunnel: [_ w343] -> w336
          frame False {
          }
          frame True {
            n143 = call-poly "Build Message with Arguments++.vi"("State With Arguments"="AsyncMessageWithoutReply", "Arguments (\"\")"="123456789" ("Arguments (\"\")"), "Target Module (\"\")"=w345) -> ("CSM Message String"=w343:string)  [unwired: 12 in]
          }
        }
        n144 = call <vilib>:"Add State(s) to Queue__JKI_lib_State_Machine.vi"("State(s) in Front (\"\")"=w336, "State(s) in (\"\")"=w337) -> ("States Out"=w338:string)  [unwired: 13 in]
      }
      frame "API: Test AsyncMessageWithoutReply via API" {
        n145 = call "CSM - Check If Module Exists.vi"("CSM Name"=w354) -> ("error out"=w349:errorcluster, "Exist?"=w350:bool, "CSM Name (Dup)"=w353:string)  [unwired: 8 in]
        n146 = case shown="True" w350 {
          tunnel: w353 -> [_ w357]
          tunnel: w348 -> [_ w360]
          tunnel: [_ w356] -> w346
          frame False {
          }
          frame True {
            n147 = call "CSM - Wait and Post Message.vi"("State"="AsyncMessageWithoutReply" ("State With Arguments"), "Current Module (\"\" to Generate an ID)"=w360, "Arguments (\"\")"="123456789" ("Arguments (\"\")"), "Target Module"=w357) -> ("error out"=w356:errorcluster)  [unwired: 11 in]
          }
        }
        n148 = call <vilib>:"Add State(s) to Queue__JKI_lib_State_Machine.vi"("State(s) in (\"\")"=w351) -> ("States Out"=w352:string)  [unwired: 14 in]
        n149 = Merge Errors(w346, w349) -> (w347:errorcluster)
      }
      frame "API: Test Argument" {
        n150 = call "uuid.vi"() -> ("UUID"=w366:string)  [unwired: 11 in]
        n151 = call "CSM - Convert HexStr to Data.vi"("HEX String"=w370) -> ("Variant"=w368:variant, "error out"=w369:errorcluster)  [unwired: 7 in]
        n152 = Bundle("", "UUID"=w366) -> (w364:cluster{string, "UUID":string})  [unwired: 1 in]
        n153 = Variant To Data(error in=w369, type=w364, Variant=w368) -> (data=w363:cluster{string, "UUID":string}, error out=w367:errorcluster)
        n154 = Unbundle(w363) -> (w362:string, "UUID"=w361:string)
        n155 = call "CSM - Check If Module Exists.vi"("Error In"=w367, "CSM Name"=w362) -> ("error out"=w371:errorcluster, "Exist?"=w372:bool, "CSM Name (Dup)"=w376:string)  [unwired: 7 in]
        n156 = case shown="True" w372 {
          tunnel: w376 -> [_ w380]
          tunnel: [_ w379] -> w373
          tunnel: w361 -> [_ w378]
          frame False {
          }
          frame True {
            n157 = call "Build Synchronous Message with Arguments.vi"("State With Arguments"="ArgumentTest", "Arguments (\"\")"=w378, "Target Module (\"\")"=w380) -> ("CSM Message String"=w379:string)  [unwired: 12 in]
          }
        }
        n158 = call <vilib>:"Add State(s) to Queue__JKI_lib_State_Machine.vi"("State(s) in Front (\"\")"=w373, "State(s) in (\"\")"=w374) -> ("States Out"=w375:string)  [unwired: 13 in]
      }
      frame "API: Test Response With Error" {
        n159 = call "CSM - Check If Module Exists.vi"("CSM Name"=w388) -> ("error out"=w382:errorcluster, "Exist?"=w383:bool, "CSM Name (Dup)"=w387:string)  [unwired: 8 in]
        n160 = case shown="True" w383 {
          tunnel: w387 -> [_ w391]
          tunnel: [_ w390] -> w384
          frame False {
          }
          frame True {
            n161 = call "uuid.vi"() -> ("UUID"=w392:string)  [unwired: 11 in]
            n162 = call "Build Synchronous Message with Arguments.vi"("State With Arguments"="Response With Error", "Arguments (\"\")"=w392, "Target Module (\"\")"=w391) -> ("CSM Message String"=w390:string)  [unwired: 12 in]
          }
        }
        n163 = call <vilib>:"Add State(s) to Queue__JKI_lib_State_Machine.vi"("State(s) in Front (\"\")"=w384, "State(s) in (\"\")"=w385) -> ("States Out"=w386:string)  [unwired: 13 in]
      }
      frame "API: Test MacroWithSubMessages" {
        n164 = call <vilib>:"Build State String with Arguments__JKI_lib_State_Machine.vi"("Arguments (\"\")"=w395, "State"="Macro: Test MacroWithSubMessages") -> ("State with Arguments"=w394:string)  [unwired: 4 in]
        n165 = call <vilib>:"Add State(s) to Queue__JKI_lib_State_Machine.vi"("State(s) in Front (\"\")"=w394, "State(s) in (\"\")"=w398) -> ("States Out"=w397:string)  [unwired: 13 in]
      }
      frame "API: Test MacroWithSubAndPostMessages" {
        n166 = call <vilib>:"Build State String with Arguments__JKI_lib_State_Machine.vi"("Arguments (\"\")"=w402, "State"="Macro: Test MacroWithSubAndPostMessages") -> ("State with Arguments"=w401:string)  [unwired: 4 in]
        n167 = call <vilib>:"Add State(s) to Queue__JKI_lib_State_Machine.vi"("State(s) in Front (\"\")"=w401, "State(s) in (\"\")"=w405) -> ("States Out"=w404:string)  [unwired: 13 in]
      }
      frame "API: Test MacroWithNonLocalSubMessages" {
        n168 = call <vilib>:"Build State String with Arguments__JKI_lib_State_Machine.vi"("Arguments (\"\")"=w409, "State"="Macro: TestMacroWithNonLocalSubMessages") -> ("State with Arguments"=w408:string)  [unwired: 4 in]
        n169 = call <vilib>:"Add State(s) to Queue__JKI_lib_State_Machine.vi"("State(s) in Front (\"\")"=w408, "State(s) in (\"\")"=w412) -> ("States Out"=w411:string)  [unwired: 13 in]
      }
      frame "API: Test Register State" {
        n170 = call <vilib>:"Build State String with Arguments__JKI_lib_State_Machine.vi"("Arguments (\"\")"=w416, "State"="Test Status") -> ("State with Arguments"=w415:string)  [unwired: 4 in]
        n171 = call <vilib>:"Add State(s) to Queue__JKI_lib_State_Machine.vi"("State(s) in Front (\"\")"=w415, "State(s) in (\"\")"=w419) -> ("States Out"=w418:string)  [unwired: 13 in]
      }
      frame "API: Test Register State Argument Info" {
        n172 = call <vilib>:"Build State String with Arguments__JKI_lib_State_Machine.vi"("Arguments (\"\")"=w423, "State"="Register State Argument Info") -> ("State with Arguments"=w422:string)  [unwired: 4 in]
        n173 = call <vilib>:"Add State(s) to Queue__JKI_lib_State_Machine.vi"("State(s) in Front (\"\")"=w422, "State(s) in (\"\")"=w426) -> ("States Out"=w425:string)  [unwired: 13 in]
      }
      frame "API: Test Register Status" {
        n174 = call <vilib>:"Build State String with Arguments__JKI_lib_State_Machine.vi"("Arguments (\"\")"=w430, "State"="Register Status") -> ("State with Arguments"=w429:string)  [unwired: 4 in]
        n175 = call <vilib>:"Add State(s) to Queue__JKI_lib_State_Machine.vi"("State(s) in Front (\"\")"=w429, "State(s) in (\"\")"=w433) -> ("States Out"=w432:string)  [unwired: 13 in]
      }
      frame "API: Test Register Interrupt" {
        n176 = call <vilib>:"Build State String with Arguments__JKI_lib_State_Machine.vi"("Arguments (\"\")"=w437, "State"="Register Interrupt") -> ("State with Arguments"=w436:string)  [unwired: 4 in]
        n177 = call <vilib>:"Add State(s) to Queue__JKI_lib_State_Machine.vi"("State(s) in Front (\"\")"=w436, "State(s) in (\"\")"=w440) -> ("States Out"=w439:string)  [unwired: 13 in]
      }
      frame "API: Test Register Status Argument Info" {
        n178 = call <vilib>:"Build State String with Arguments__JKI_lib_State_Machine.vi"("Arguments (\"\")"=w444, "State"="Register Status Argument Info") -> ("State with Arguments"=w443:string)  [unwired: 4 in]
        n179 = call <vilib>:"Add State(s) to Queue__JKI_lib_State_Machine.vi"("State(s) in Front (\"\")"=w443, "State(s) in (\"\")"=w447) -> ("States Out"=w446:string)  [unwired: 13 in]
      }
      frame "API: Test Status A" {
        n180 = call <vilib>:"Build State String with Arguments__JKI_lib_State_Machine.vi"("Arguments (\"\")"=w451, "State"="Broadcast Status A") -> ("State with Arguments"=w452:string)  [unwired: 4 in]
        n181 = call <vilib>:"Add State(s) to Queue__JKI_lib_State_Machine.vi"("State(s) in Front (\"\")"=w452, "State(s) in (\"\")"=w454) -> ("States Out"=w453:string)  [unwired: 13 in]
      }
      frame "API: Test State A" {
        n182 = call <vilib>:"Build State String with Arguments__JKI_lib_State_Machine.vi"("Arguments (\"\")"=w458, "State"="State A") -> ("State with Arguments"=w459:string)  [unwired: 4 in]
        n183 = call <vilib>:"Add State(s) to Queue__JKI_lib_State_Machine.vi"("State(s) in Front (\"\")"=w459, "State(s) in (\"\")"=w461) -> ("States Out"=w460:string)  [unwired: 13 in]
      }
      frame "API: Test State B" {
        n184 = call <vilib>:"Build State String with Arguments__JKI_lib_State_Machine.vi"("Arguments (\"\")"=w465, "State"="State B") -> ("State with Arguments"=w466:string)  [unwired: 4 in]
        n185 = call <vilib>:"Add State(s) to Queue__JKI_lib_State_Machine.vi"("State(s) in Front (\"\")"=w466, "State(s) in (\"\")"=w468) -> ("States Out"=w467:string)  [unwired: 13 in]
      }
      frame "API: Test Status B" {
        n186 = call <vilib>:"Build State String with Arguments__JKI_lib_State_Machine.vi"("Arguments (\"\")"=w472, "State"="Broadcast Status B") -> ("State with Arguments"=w473:string)  [unwired: 4 in]
        n187 = call <vilib>:"Add State(s) to Queue__JKI_lib_State_Machine.vi"("State(s) in Front (\"\")"=w473, "State(s) in (\"\")"=w475) -> ("States Out"=w474:string)  [unwired: 13 in]
      }
      frame "API: Local Registration" {
        # "Test Status @ From >> Handler Message @ To -><register>"
        n188 = call "Strip CSM name.vi"("CSM name"=w483) -> ("error out"=w481:errorcluster, "CSM name core"=w478:string)  [unwired: 7 in, 2 out]
        n189 = call-poly "Build Message with Arguments++.vi"("Target CSM"=w479, "Source CSM (* as Default)"=w478, "Status"="Test Status", "API (If \"\", Same As \"Status\")"="Handler Message") -> ("CSM Message String"=w480:string)  [unwired: 11 in]
        n190 = call <vilib>:"Add State(s) to Queue__JKI_lib_State_Machine.vi"("State(s) in Front (\"\")"=w480, "State(s) in (\"\")"=w487) -> ("States Out"=w486:string)  [unwired: 13 in]
      }
      frame "API: Local Registration II" {
        # "Test Status @ From >> Handler Message -><register>"
        n191 = call "Strip CSM name.vi"("CSM name"=w492) -> ("error out"=w490:errorcluster, "CSM name core"=w488:string)  [unwired: 7 in, 2 out]
        n192 = call-poly "Build Message with Arguments++.vi"("Source CSM (* as Default)"=w488, "Status"="Test Status", "API (If \"\", Same As \"Status\")"="Handler Message") -> ("CSM Message String"=w489:string)  [unwired: 12 in]
        n193 = call <vilib>:"Add State(s) to Queue__JKI_lib_State_Machine.vi"("State(s) in Front (\"\")"=w489, "State(s) in (\"\")"=w496) -> ("States Out"=w495:string)  [unwired: 13 in]
      }
      frame "API: Local Unregistration" {
        # "Test Status @ From >> Handler Message @ To -><unregister>"
        n194 = call "Strip CSM name.vi"("CSM name"=w502) -> ("error out"=w500:errorcluster, "CSM name core"=w497:string)  [unwired: 7 in, 2 out]
        n195 = call-poly "Build Message with Arguments++.vi"("Target CSM"=w498, "Source CSM (* as Default)"=w497, "Status"="Test Status", "API (If \"\", Same As \"Status\")"="Handler Message") -> ("CSM Message String"=w499:string)  [unwired: 11 in]
        n196 = call <vilib>:"Add State(s) to Queue__JKI_lib_State_Machine.vi"("State(s) in Front (\"\")"=w499, "State(s) in (\"\")"=w506) -> ("States Out"=w505:string)  [unwired: 13 in]
      }
      frame "API: Local Registration via API" {
        # "Test Status @ From >> Handler Message @ To -><register>"
        n197 = call "Strip CSM name.vi"("CSM name"=w513) -> ("error out"=w512:errorcluster, "CSM name core"=w508:string)  [unwired: 7 in, 2 out]
        n198 = call "CSM - Register Broadcast.vi"("CSM Name(Empty for Broadcast Event)"=w507, "Source CSM Name (* as Default)"=w508, "Trigger"="Test Status", "API (If \"\", Same as Trigger)"="Handler Message", "Error In"=w512) -> ("error out"=w511:errorcluster)  [unwired: 9 in, 1 out]
        n199 = call <vilib>:"Add State(s) to Queue__JKI_lib_State_Machine.vi"("State(s) in (\"\")"=w516) -> ("States Out"=w515:string)  [unwired: 14 in]
      }
      frame "API: Local Unregistration via API" {
        # "Test Status @ From >> Handler Message @ To -><unregister>"
        n200 = call "Strip CSM name.vi"("CSM name"=w523) -> ("error out"=w522:errorcluster, "CSM name core"=w518:string)  [unwired: 7 in, 2 out]
        n201 = call "CSM - Unregister Broadcast.vi"("CSM Name(Empty for Broadcast Event)"=w517, "Source CSM Name (* as Default)"=w518, "Trigger"="Test Status", "API (\"*\" as Default)"="Handler Message", "Error In"=w522) -> ("error out"=w521:errorcluster)  [unwired: 9 in, 1 out]
        n202 = call <vilib>:"Add State(s) to Queue__JKI_lib_State_Machine.vi"("State(s) in (\"\")"=w526) -> ("States Out"=w525:string)  [unwired: 14 in]
      }
      frame "API: API2" {
        # "#CSM API Example\nCopy/Rename this case for your own API"
        # "unpack Hex String  to Variant\nif complex parameter is needed."
        n203 = call "CSM - Convert HexStr to Data.vi"("HEX String"=w528) -> ()  [unwired: 7 in, 2 out]
        n204 = disable-structure shown="Enabled" {
          disable-tunnel: [w531 "API2 Response"] -> w527
          frame Disabled {
            # "pack variant to hexstr \nif complex response is needed."
            # "complex Response"
            n205 = call "CSM - Convert Data to HexStr.vi"() -> ("HEX String (0-9,A-F)"=w531:string)  [unwired: 9 in]
          }
          frame Enabled {
          }
        }
      }
      frame "---------- Action ----------" {
        # "#CSM \"Category Seperator\"\nDo not put any code in this frame."
        n206 = call <vilib>:"Add State(s) to Queue__JKI_lib_State_Machine.vi"("State(s) in (\"\")"=w535) -> ("States Out"=w534:string)  [unwired: 14 in]
      }
      frame "Action: action1" {
        # "#CSM \"Internal State\"\nThis category is used for holding internal states"
        n207 = call <vilib>:"Add State(s) to Queue__JKI_lib_State_Machine.vi"("State(s) in (\"\")"=w538) -> ("States Out"=w537:string)  [unwired: 14 in]
      }
      frame "Test Status" {
        n208 = call <vilib>:"Add State(s) to Queue__JKI_lib_State_Machine.vi"("State(s) in (\"\")"=w542) -> ("States Out"=w541:string)  [unwired: 14 in]
      }
      frame "Register State Argument Info" {
        n209 = call "Strip CSM name.vi"("CSM name"=w546) -> ("error out"=w545:errorcluster, "CSM name core"=w547:string)  [unwired: 7 in, 2 out]
        n210 = Concatenate Strings(w543, "+", w547) -> (w544:string)
        n211 = call <vilib>:"Add State(s) to Queue__JKI_lib_State_Machine.vi"("State(s) in (\"\")"=w549) -> ("States Out"=w551:string)  [unwired: 14 in]
      }
      frame "Register Status" {
        n212 = call <vilib>:"Build State String with Arguments__JKI_lib_State_Machine.vi"("Arguments (\"\")"=w552, "State"="Test Status") -> ("State with Arguments"=w554:string)  [unwired: 4 in]
        n213 = call "CSM - Broadcast Status Change.vi"("Status With Arguments"=w554, "State Queue"=w556) -> ("Remaining States"=w553:string)  [unwired: 13 in]
      }
      frame "Register Interrupt" {
        n214 = call-poly "Build Message with Arguments++.vi"("State With Arguments"="Test Interrupt", "Arguments (\"\")"=w561) -> ("CSM Message String"=w560:string)  [unwired: 13 in]
        n215 = call <vilib>:"Add State(s) to Queue__JKI_lib_State_Machine.vi"("State(s) in Front (\"\")"=w560, "State(s) in (\"\")"=w559) -> ("States Out"=w558:string)  [unwired: 13 in]
      }
      frame "Register Status Argument Info" {
        w569 = "Test Status Argument Info"
        n216 = call "Strip CSM name.vi"("CSM name"=w567) -> ("error out"=w565:errorcluster, "CSM name core"=w566:string)  [unwired: 7 in, 2 out]
        n217 = Concatenate Strings(w569, "+", w566) -> (w564:string)
        n218 = call <vilib>:"Build State String with Arguments__JKI_lib_State_Machine.vi"("Arguments (\"\")"=w564, "State"=w569) -> ("State with Arguments"=w571:string)  [unwired: 4 in]
        n219 = call "CSM - Broadcast Status Change.vi"("Status With Arguments"=w571, "State Queue"=w572) -> ("Remaining States"=w570:string)  [unwired: 13 in]
      }
      frame "Broadcast Status A" {
        n220 = call <vilib>:"Build State String with Arguments__JKI_lib_State_Machine.vi"("Arguments (\"\")"=w574, "State"="Status A") -> ("State with Arguments"=w576:string)  [unwired: 4 in]
        n221 = call "CSM - Broadcast Status Change.vi"("Status With Arguments"=w576, "State Queue"=w578) -> ("Remaining States"=w575:string)  [unwired: 13 in]
      }
      frame "Broadcast Status B" {
        n222 = call <vilib>:"Build State String with Arguments__JKI_lib_State_Machine.vi"("Arguments (\"\")"=w580, "State"="Status B") -> ("State with Arguments"=w582:string)  [unwired: 4 in]
        n223 = call "CSM - Broadcast Status Change.vi"("Status With Arguments"=w582, "State Queue"=w584) -> ("Remaining States"=w581:string)  [unwired: 13 in]
      }
      frame "State A" {
        n224 = call <vilib>:"Add State(s) to Queue__JKI_lib_State_Machine.vi"("State(s) in (\"\")"=w588) -> ("States Out"=w587:string)  [unwired: 14 in]
      }
      frame "State B" {
        n225 = call <vilib>:"Add State(s) to Queue__JKI_lib_State_Machine.vi"("State(s) in (\"\")"=w593) -> ("States Out"=w592:string)  [unwired: 14 in]
      }
      frame "Message" {
      }
      frame "SubMessage1" {
      }
      frame "SubMessage2" {
      }
      frame "SubMessage3" {
        n226 = call "Strip CSM name.vi"("CSM name"=w614) -> ("error out"=w612:errorcluster, "CSM name core"=w613:string)  [unwired: 7 in, 2 out]
        n227 = call "CSM - Set Module Attribute.vi"("CSM Name"=w613, "Attribute"=w611, "Value"=w610, "Error In"=w612) -> ("error out"=w608:errorcluster)  [unwired: 8 in, 3 out]
        n228 = Merge Errors(w608, w617) -> (w609:errorcluster)
      }
      frame "PostMessage1" {
      }
      frame "Message With Error" {
        n229 = Merge Errors(errorcluster {"status"=TRUE, "code"=1234567898, "source"="Simulated Error\nwill be sent to Response case"} ("error out"), w623) -> (w622:errorcluster)
      }
      frame "Response With Error" {
        n230 = Merge Errors(errorcluster {"status"=TRUE, "code"=1234567898, "source"="Simulated Error"} ("error out"), w629) -> (w628:errorcluster)
      }
      frame "ArgumentTest" {
        n231 = call "Strip CSM name.vi"("CSM name"=w640) -> ("error out"=w637:errorcluster, "CSM name core"=w639:string)  [unwired: 7 in, 2 out]
        n232 = call "CSM - Set Module Attribute.vi"("CSM Name"=w639, "Attribute"=w636, "Value"=w638, "Error In"=w637) -> ("error out"=w634:errorcluster)  [unwired: 8 in, 3 out]
        n233 = Merge Errors(w634, w643) -> (w635:errorcluster)
      }
      frame "AsyncMessageWithoutReply" {
        # "123456789 string constant"
        n234 = call "Strip CSM name.vi"("CSM name"=w648) -> ("error out"=w646:errorcluster, "CSM name core"=w647:string)  [unwired: 7 in, 2 out]
        n235 = call "CSM - Set Module Attribute.vi"("CSM Name"=w647, "Attribute"=w649, "Value"=w650, "Error In"=w646) -> ("error out"=w644:errorcluster)  [unwired: 8 in, 3 out]
        n236 = Merge Errors(w644, w653) -> (w645:errorcluster)
      }
      frame "Handler Message" {
        n237 = call "Strip CSM name.vi"("CSM name"=w660) -> ("error out"=w658:errorcluster, "CSM name core"=w659:string)  [unwired: 7 in, 2 out]
        n238 = call "CSM - Set Module Attribute.vi"("CSM Name"=w659, "Attribute"=w656, "Value"=w655, "Error In"=w658) -> ("error out"=w654:errorcluster)  [unwired: 8 in, 3 out]
        n239 = Merge Errors(w663, w654) -> (w657:errorcluster)
      }
      frame "Handler Message With Counter" {
        n240 = Unbundle By Name(w669) -> ("Counter"=w670:u32)
        n241 = Decimal String To Number(string=w667) -> (number=w664:i32)  [unwired: 2 in, 1 out]
        n242 = Increment(x=w670) -> (x+1=w665:u32)
        n243 = Bundle By Name(cluster=w669, "Counter"=w665) -> (w668:T6)
        n244 = Equal?(x=w665, y=w664) -> (x = y?=w666:bool)
        n245 = call "Strip CSM name.vi"("CSM name"=w676) -> ("error out"=w674:errorcluster, "CSM name core"=w675:string)  [unwired: 7 in, 2 out]
        n246 = case shown="True" w666 {
          tunnel: w675 -> [_ w684]
          tunnel: w674 -> [w679 w683]
          tunnel: w672 -> [_ w682]
          tunnel: [w679 w681] -> w671
          tunnel: w665 -> [_ w680]
          frame False {
          }
          frame True {
            n247 = call "CSM - Set Module Attribute.vi"("CSM Name"=w684, "Attribute"=w682, "Value"=w680, "Error In"=w683) -> ("error out"=w681:errorcluster)  [unwired: 8 in, 3 out]
          }
        }
        n248 = Merge Errors(w678, w671) -> (w673:errorcluster)
      }
      frame "Reset Counter" {
        # "#CSM \"Internal State\"\nThis category is used for holding internal states"
        n249 = Bundle By Name(cluster=w687, "Counter"=u32 0) -> (w685:T6)
        n250 = call <vilib>:"Add State(s) to Queue__JKI_lib_State_Machine.vi"("State(s) in (\"\")"=w689) -> ("States Out"=w688:string)  [unwired: 14 in]
      }
    }
  }
